vi "Grab (Express).vi"() -> ()   [LabVIEW 2011]
doc: "The Grab (Express) VI acquires images continuously and displays the images in an image control using the Vision Acquisition Express VI. A grab is appropriate for high-speed applications in which you need to process only one image at a time."
uses:
  Instance           1 22Saved   Grab (Express) .vi
panel:
  out "Buffer Number":u32
  out "Image":T1(plugin-control)
  out "Frame Rate":dbl(knob) scale=0.0..100.0
  in  "Stop":bool
  # "Overview: Demonstrates\nRequirements: Vision Acquisition Software\nInstructions: Run the VI"
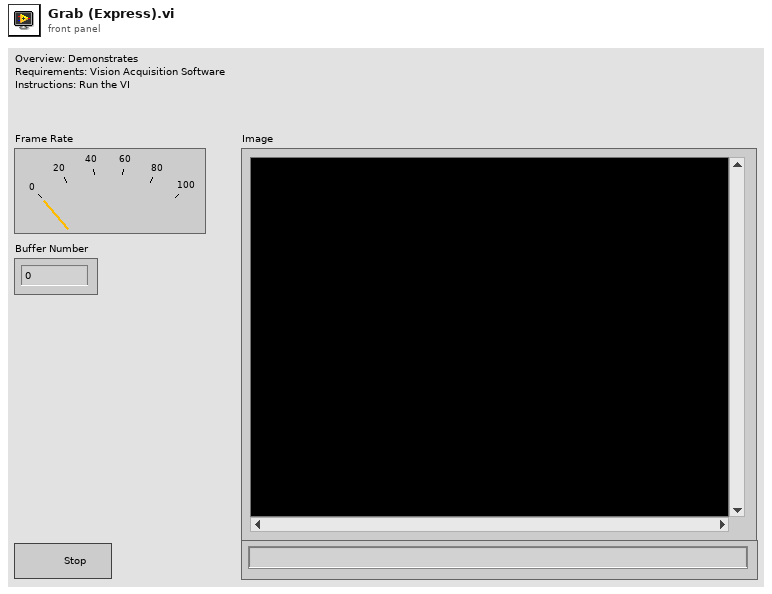
[diagram p1: front panel]
types:
  T1 = typedef "IMAQ Image.ctl" = refnum<image>
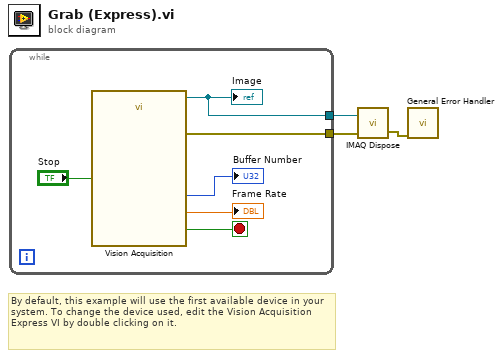
[diagram p0: block diagram]
diagram:
  # "By default, this example will use the first available device in your system. To change the device used, edit the Vision Acquisition Express VI by double clicking on it."
  n1 = while {
    tunnel: [w6] -> w3
    tunnel: [w4] -> w1
    stop <- w9 stop-if-true
    n2 = call "Vision Acquisition"("Stop (F)"="Stop") -> ("Image Out"=w4:T1, "Image Number"=→"Buffer Number":u32, "Frame Rate"=→"Frame Rate":dbl, "Stopped"=w9:bool, "error out"=w6:errorcluster)  [unwired: 1 in, 21 out]
    "Image" <- w4
  }
  n3 = call "IMAQ Dispose"("Image"=w1, "error in (no error)"=w3) -> ("error out"=w2:errorcluster)  [unwired: 4 in]
  n4 = call <vilib>:"General Error Handler.vi"("error in (no error)"=w2) -> ()  [unwired: 1 in, 14 out]
